vi "Indexer.vi"(11 "input cluster":T2) -> (3 "Indexer Info":T1)   [LabVIEW 2015]
uses:
  Joystick/ControlsToCommands.ctl
  References/Indexer Info.ctl
  References/Refnums.vi
panel:
  in  "Numeric":dbl min=-1.0 max=1.0 step=1.0
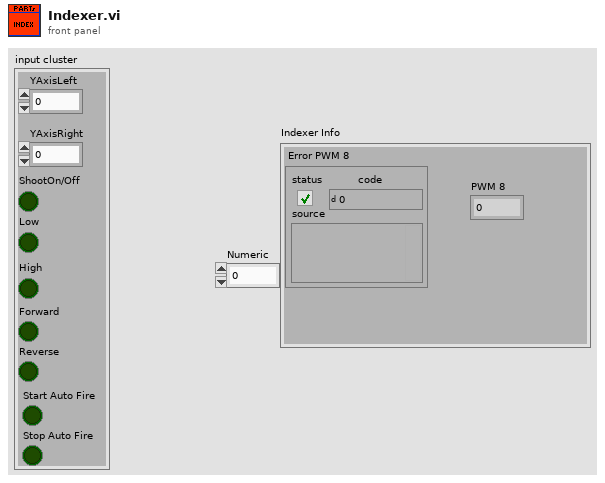
[diagram p1: front panel]
types:
  T1 = typedef "Indexer Info.ctl" = cluster{"Error PWM 8":errorcluster, "PWM 8":dbl}
  T2 = typedef "ControlsToCommands.ctl" = cluster{"YAxisLeft":dbl, "YAxisRight":dbl, "ShootOn/Off":bool, "Low":bool, "High":bool, "Forward":bool, "Reverse":bool, "Start Auto Fire":bool, "Stop Auto Fire":bool}
  T3 = typedef "WPI_MotorControlDeviceRef.ctl" = cluster{"DeviceStatus":errorcluster, "Type":T4, "PWM":cluster{"PWM Channel":T5, "DeadBand":T6}, "CAN":cluster{"Device Number":u8, "Control Mode":T7, "Semaphore":T8, "Max Vout":dbl, "TalonSRX Control Mode":T9}, "Invert":bool}
  T4 = typedef "WPI_MotorControlType.ctl" = enum16{"PWM", "CAN", "CANTalonSRX"}
  T5 = typedef "FPGA_DIOPWMChannel.ctl" = enum8{"PWM 0", "PWM 1", "PWM 2", "PWM 3", "PWM 4", "PWM 5", "PWM 6", "PWM 7", "PWM 8", "PWM 9", "PWM MXP 0", "PWM MXP 1", "PWM MXP 2", "PWM MXP 3", "PWM MXP 4", "PWM MXP 5", "PWM MXP 6", "PWM MXP 7", "PWM MXP 8", "PWM MXP 9", "Invalid"}
  T6 = typedef "WPI_PWMDeadband.ctl" = cluster{"Name":string, "maxPositivePwm":i32, "minPositivePwm":i32, "centerPwm":i32, "maxNegativePwm":i32, "minNegativePwm":i32, "angularRange":u16}
  T7 = typedef "WPI_CANJaguar_ControlMode.ctl" = enum8{"Percent VBus", "Current", "Speed", "Position", "Voltage"}
  T8 = typedef "Semaphore RefNum" = refnum<k1>
  T9 = typedef "WPI_CANTalonSRX_APIControlMode.ctl" = enum8{"Percent VBus", "Speed", "Position", "Slave", "Unchanged / Invalid", "Voltage Compensation", "Current", "Motion Profile"}
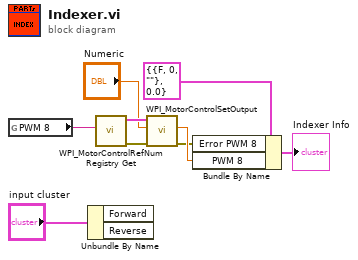
[diagram p0: block diagram]
diagram:
  n1 = global read "Refnums.vi" "PWM 8"() -> (w8:string)
  n2 = Unbundle By Name("input cluster") -> ()  [unwired: 2 out]
  n3 = call <vilib>:"WPI_MotorControlRefNum Registry Get.vi"("refnum name"=w8) -> ("error out"=w6:errorcluster, "MotorControlDevRef"=w7:T3)  [unwired: 9 in]
  n4 = call <vilib>:"WPI_MotorControlSetOutput.vi"("error in (no error)"=w6, "Output"="Numeric", "MotorControlDevRef"=w7) -> ("error out"=w3:errorcluster, "Motor Output"=w4:dbl)  [unwired: 6 in, 1 out]
  n5 = Bundle By Name(cluster=T1 {"Error PWM 8"={"status"=FALSE, "code"=0, "source"=""}, "PWM 8"=0.0} ("Indexer Info"), "Error PWM 8"=w3, "PWM 8"=w4) -> (→"Indexer Info":T1)
